vi "Enqueue Null Command.vi"(10 "NewVal":bool, 11 "Queue in":refnum<queue>) -> ()   [LabVIEW 2020]
uses:
  Type Definitions/Payload Class.ctl
  Type Definitions/Enum - Commands.ctl
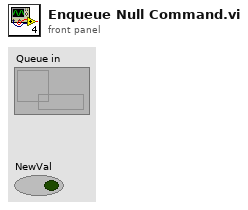
[diagram p1: front panel]
types:
  T1 = typedef "Enum - Commands.ctl" = enum16{"Null", "Analog Output Command", "Digital Output Command"}
  T2 = typedef "Payload Class.ctl" = enum16{"System State", "Parameters", "Metadata", "Software Monitor", "Data", "Commands"}
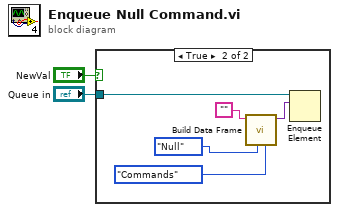
[diagram p0: block diagram]
diagram:
  n1 = case shown="True" "NewVal" {
    tunnel: "Queue in" -> [_ w7]
    frame False {
    }
    frame True {
      n2 = call "Build Data Frame.vi"("Payload Class (Data)"=Payload_Class."Commands", "Payload ID (0)"=Enum_-_Commands."Null" ("Commands"), "Payload (Empty String)"="") -> ("Frame"=w6:variant)  [unwired: 7 in, 1 out]
      n3 = Enqueue Element(queue=w7, element=w6) -> ()  [unwired: 2 in, 3 out]
    }
  }
